vi "Read (Str).vi"(6 "ISOBUS address":T2=-1 caption="ISOBUS address (-1)", 8 "error in":errorcluster, 10 "SCPI Message(s)":string[](array[string]), 11 "Mercury Reference In":T3) -> (0 "error out":errorcluster, 2 "Response":string, 3 "Mercury Reference Out":T3, 4 "Valid?":T1)   [LabVIEW 2019, in "Mercury iXX.lvlib"]
doc: "Read the response from the instrument and outputs the result as a string indicator."
uses:
  Mercury iXX.lvlib
  Public/Controls/Mercury Reference.ctl
  Public/Controls/Comms Transport Layer.ctl
  Controls/Query Dynamic Reference.ctl
  Public/Controls/ISOBus Address.ctl
  Public/Controls/Is Valid LED.ctl
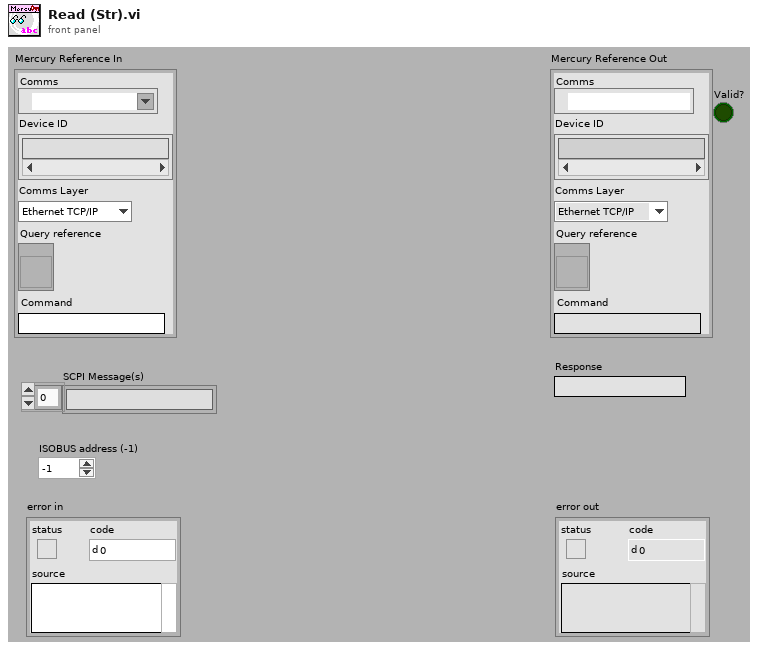
[diagram p1: front panel]
types:
  T1 = typedef "Mercury iXX.lvlib/Is Valid LED.ctl" = bool
  T2 = typedef "Mercury iXX.lvlib/ISOBus Address.ctl" = i32
  T3 = typedef "Mercury iXX.lvlib/Mercury Reference.ctl" = cluster{"Comms":refnum<visa-resource-name>, "Device ID":string[], "Comms Layer":T4, "Command":string, "Query reference":T5}
  T4 = typedef "Mercury iXX.lvlib/Comms Transport Layer.ctl" = enum16{"Ethernet TCP/IP", "USB", "ISOBus - RS-232", "GPIB"}
  T5 = typedef "Mercury iXX.lvlib/Query Dynamic Reference.ctl" = refnum<vi>
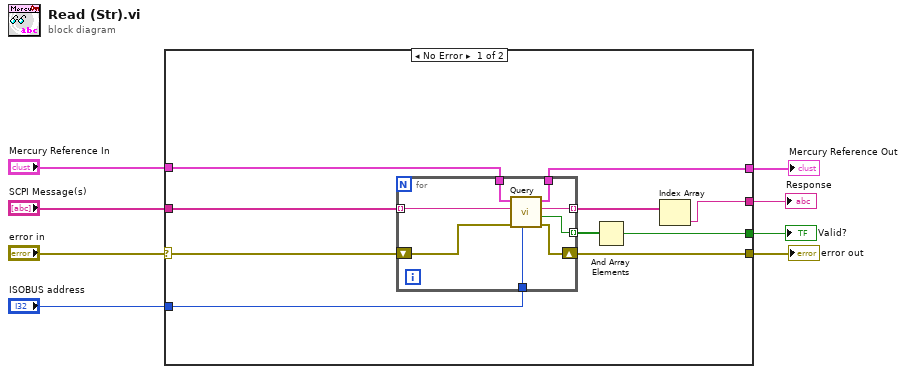
[diagram p0: block diagram]
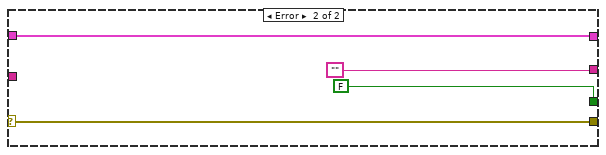
[diagram p2: hidden frame]
diagram:
  n1 = case shown="No Error" "error in" {
    selector: "error in" -> [w16 w29]
    tunnel: "Mercury Reference In" -> [w18 w30]
    tunnel: [w17 w30] -> w7
    tunnel: [w15 w29] -> w6
    tunnel: "ISOBUS address" -> [w10 _]
    tunnel: [w11 ""] -> w3
    tunnel: [w13 FALSE ("Valid?")] -> w2
    tunnel: "SCPI Message(s)" -> [w9 _]
    frame No Error {
      n2 = for {
        tunnel: [w26] -> w12 mode=indexing
        tunnel: w18 -> [w25]
        tunnel: [w24] -> w17
        shift-right: [w22] -> w15
        shift-left: w16 -> [w23]
        tunnel: [w21] -> w14 mode=indexing
        tunnel: w10 -> [w20]
        tunnel: w9 -> [w19] mode=indexing
        n3 = call "Query.vi"("ISOBUS address"=w20, "error in"=w23, "Command"=w19, "Mercury Reference In"=w25) -> ("error out"=w22:errorcluster, "Valid?"=w21:bool, "Data"=w26:string, "Mercury Reference Out"=w24:T3)  [unwired: 1 in, 3 out]
      }
      n4 = And Array Elements(Boolean array=w14) -> (logical AND=w13:bool)
      n5 = Index Array(array=w12) -> (element=w11:string)  [unwired: 1 in]
    }
    frame Error {
    }
  }
  "Mercury Reference Out" <- w7
  "error out" <- w6
  "Response" <- w3
  "Valid?" <- w2
